vi "Close connection.vi"(8 "error in (no error)":errorcluster, 11 "TCP Writer in":refnum<class "TCP Writer.lvclass">) -> (0 "error out":errorcluster, 3 "TCP Writer out":refnum<class "TCP Writer.lvclass">)   [LabVIEW 2026, in "TALOS.lvlib" / "TCP Writer.lvlib" / "TCP Writer.lvclass"]
uses:
  TCP Writer.lvclass
  Ancestor/Ancestor/Infinite Message Selector.ctl
  TCP Writer Consumer Case Selector.ctl
  TCP Writer.lvclass/TCP Writer.ctl
  Ancestor/Ancestor/Ancestor.lvclass
  TALOS.lvlib
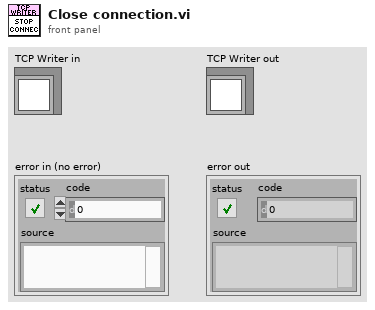
[diagram p1: front panel]
types:
  T1 = typedef "TALOS.lvlib/TCP Writer.lvlib/TCP Writer.lvclass/TCP Writer Consumer Case Selector.ctl" = enum16{"Send message", "Idle", "Check Connection", "Open connection", "Set Client ID"}
  T2 = typedef "TALOS.lvlib/Ancestor.lvlib/Ancestor.lvclass/Infinite Message Selector.ctl" = enum16{"Start", "Stop", "Check", "Flush (Stop all)", "Init"}
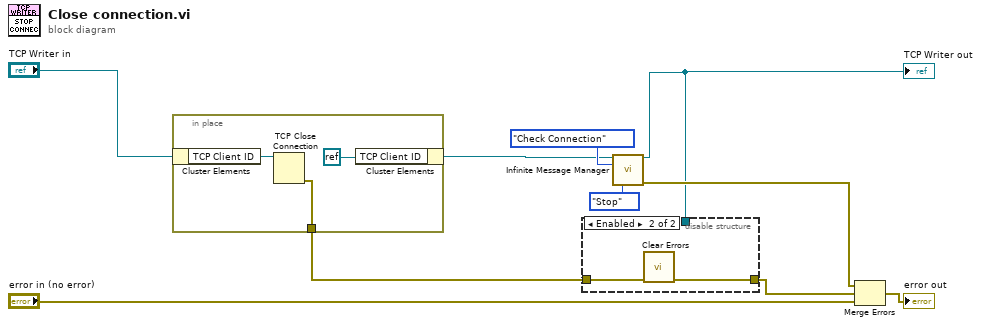
[diagram p0: block diagram]
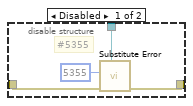
[diagram p2: hidden frame]
diagram:
  n1 = in-place {
    in-place-border: [w13] -> w3
    n2 = in-place-cluster #1("TCP Writer in") -> ("TCP Client ID"=w12:refnum<k5>)
    n3 = TCP Close Connection(connection ID=w12) -> (error out=w13:errorcluster)  [unwired: 2 in, 1 out]
    n4 = in-place-cluster #1("TCP Client ID"=refnum<k0> refnum) -> (w1:refnum<class "TCP Writer.lvclass">)
  }
  n5 = call-dynamic "Infinite Message Manager.vi"("Father of all uServices in"=w1, "Consumer Case Selector"=TCP_Writer_Consumer_Case_Selector."Check Connection" ("TCP Writer Consumer Case Selector"), "Infinite Message Selector"=Infinite_Message_Selector."Stop") -> ("Father of all uServices out"=w5:refnum<class "TCP Writer.lvclass">, "error out"=w10:errorcluster)  [unwired: 10 in, 1 out]
  "TCP Writer out" <- w5
  n6 = disable-structure shown="Enabled" {
    disable-tunnel: [w17 w18] -> w6
    disable-tunnel: w5 -> [w16 _]
    disable-tunnel: w3 -> [w14 w19]
    frame Disabled {
      # "#5355"
      n7 = call "Substitute Error.vi"("LabVIEW Object"=w16, "error in (no error)"=w14, "Error Code"=5355) -> ("error out"=w17:errorcluster)  [unwired: 8 in]
    }
    frame Enabled {
      n8 = call <vilib>:"Clear Errors.vi"("error in (no error)"=w19) -> ("error out"=w18:errorcluster)  [unwired: 5 in, 1 out]
    }
  }
  n9 = Merge Errors(w10, w6, "error in (no error)") -> (→"error out":errorcluster)
